vi "configure input.vi"(8 "error in (no error)":errorcluster, 9 "InputMode":u32(ring) items=["DC_HighImp", "DC_LowImp", "AC_Slow", "AC_Fast"], 10 "Board":u16, 11 "identifier":string) -> (0 "error out":errorcluster, 3 "function return":u32)   [LabVIEW 2015, in "XGL_DPP.lvlib"]
doc: "EXTERN DECLSPEC uint32_t CALL_CONV configure_input(const char * identifier, uint16_t Board, const InputMode InputMode);"
uses:
  XGL_DPP.lvlib
  XGL_DPP.dll
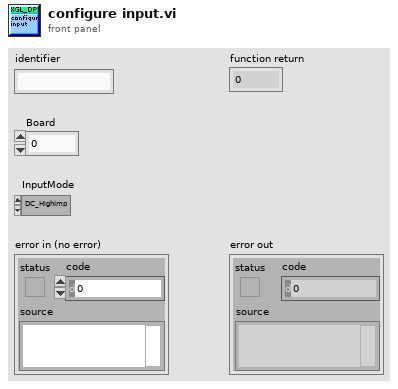
[diagram p1: front panel]
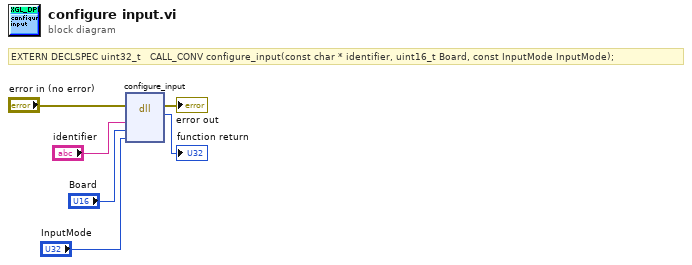
[diagram p0: block diagram]
diagram:
  # "EXTERN DECLSPEC uint32_t   CALL_CONV configure_input(const char * identifier, uint16_t Board, const InputMode InputMode);"
  n1 = dll-call lib="D:/Users/XRF/Desktop/Scanning Software_Demokritos_2015_v7/libs/Vis_2/XGL_DPP.*" fn="configure_input"(error in="error in (no error)", "identifier"="identifier", "Board"="Board", "InputMode"="InputMode") -> (error out=→"error out":errorcluster, →"function return":u32)  [unwired: 5 in, 1 out]
